vi "Write Amphipods.vi"(8 "error in (no error)":errorcluster, 10 "Amphipods":refnum<class "Amphipod.lvclass">[](array[class]), 11 "Burrow in":refnum<class "Burrow.lvclass">) -> (0 "error out":errorcluster, 3 "Burrow out":refnum<class "Burrow.lvclass">)   [LabVIEW 2019, in "23.lvlib" / "Burrow.lvclass"]
uses:
  Burrow.lvclass
  Amphipod/Amphipod.lvclass
  Burrow.lvclass/Burrow.ctl
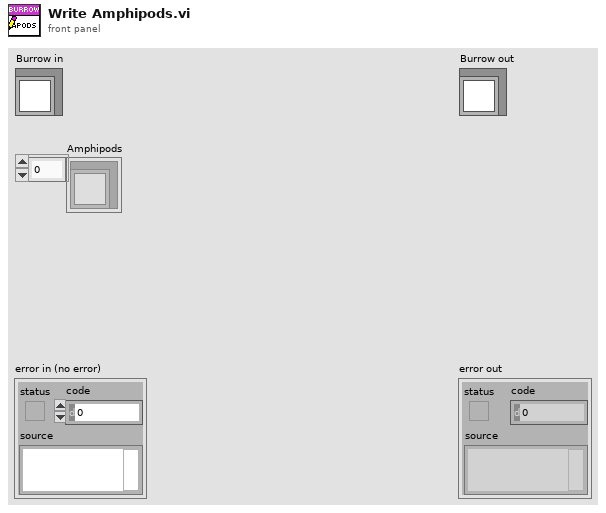
[diagram p1: front panel]
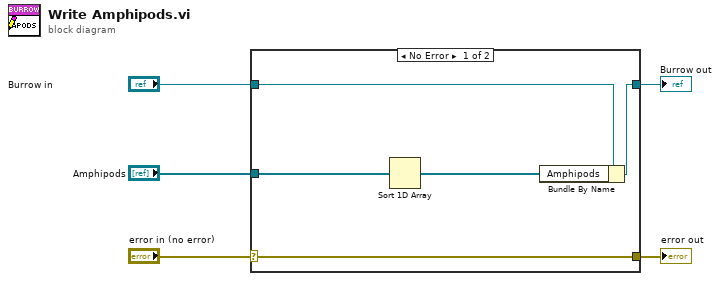
[diagram p0: block diagram]
diagram:
  n1 = case shown="No Error" "error in (no error)" {
    selector: "error in (no error)" -> [w10 w11]
    tunnel: [w10 w11] -> w4
    tunnel: [w8 w12] -> w2
    tunnel: "Burrow in" -> [w9 w12]
    tunnel: "Amphipods" -> [w6 _]
    frame No Error {
      n2 = Sort 1D Array(array=w6) -> (sorted array=w7:refnum<class "Amphipod.lvclass">[])
      n3 = Bundle By Name(cluster=w9, "Amphipods"=w7) -> (w8:refnum<class "Burrow.lvclass">)
    }
    frame Error {
    }
  }
  "error out" <- w4
  "Burrow out" <- w2
